vi "Config (SubVI).vi"() -> (2 "Config Data":T1, 3 "Scale Data":T2)   [LabVIEW 2014]
panel:
  in  "stop":bool
  in  "Config Data 2":T1={"Sample Rate"=1000.0, "Number of Channels"=1}
  in  "Scale Data 2":T2={"TDX"={"Range"=1.0}, "Encoder"={"Ratio"=1.0}}
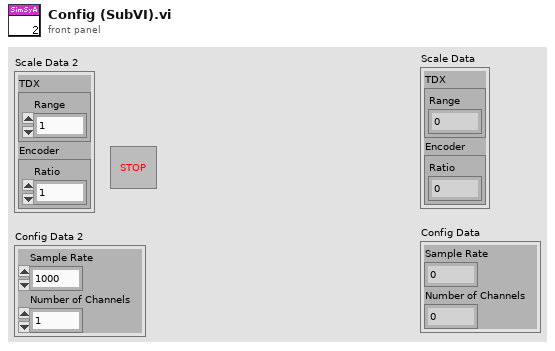
[diagram p1: front panel]
types:
  T1 = cluster{"Sample Rate":sgl, "Number of Channels":u64}
  T2 = cluster{"TDX":cluster{"Range":sgl}, "Encoder":cluster{"Ratio":sgl}}
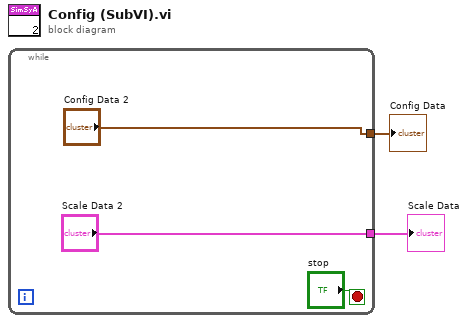
[diagram p0: block diagram]
diagram:
  n1 = while {
    tunnel: ["Scale Data 2"] -> w2
    tunnel: ["Config Data 2"] -> w1
    stop <- "stop" stop-if-true
  }
  "Scale Data" <- w2
  "Config Data" <- w1
